vi "Engine Config Cluster to DSF Config File.vi"(8 "error in (no error)":errorcluster, 10 "dsf configuration file path":path, 11 "input cluster":T1) -> (0 "error out":errorcluster)   [LabVIEW 2017, in "Data Sharing Framework Core.lvlib" / "Data Sharing Framework Engine.lvlib"]
uses:
  Data Sharing Framework Engine.lvlib
  Configuration/1.0.0/Public/Controls/DSF Engine Framework Configuration.ctl
  Configuration/1.0.0/Public/Controls/DSF Engine Plugin Configuration.ctl
  Configuration/1.0.0/Public/Controls/DSF Timing Info.ctl
  Configuration/1.0.0/Public/Controls/DSF Engine Transfer Group Configuration.ctl
  Configuration/1.0.0/Public/Controls/DSF Direction.ctl
  Configuration/1.0.0/Public/Controls/DSF Engine Transfer Configuration.ctl
  Configuration/1.0.0/Public/Controls/DSF Byte Order.ctl
  Configuration/1.0.0/Public/Controls/DSF Engine Channel Configuration.ctl
  Configuration/1.0.0/Public/Controls/DSF Data Type.ctl
  Configuration/1.0.0/Public/Controls/DSF Settings Info.ctl
  Configuration/1.0.0/Public/Controls/DSF Plugin Info.ctl
  Configuration/1.0.0/Public/Controls/DSF Group Info.ctl
  Configuration/1.0.0/Public/Controls/DSF Transfer Info.ctl
  Configuration/1.0.0/Public/Controls/DSF Channel Info.ctl
  Configuration/1.0.0/Public/Write Item/Write Channel.vi
  Configuration/1.0.0/Public/Write Item/Write Transfer.vi
  Configuration/1.0.0/Public/Write Item/Write Group.vi
  Configuration/1.0.0/Public/Write Item/Write Plugin.vi
  Configuration/1.0.0/Data Sharing Framework Configuration.lvlib
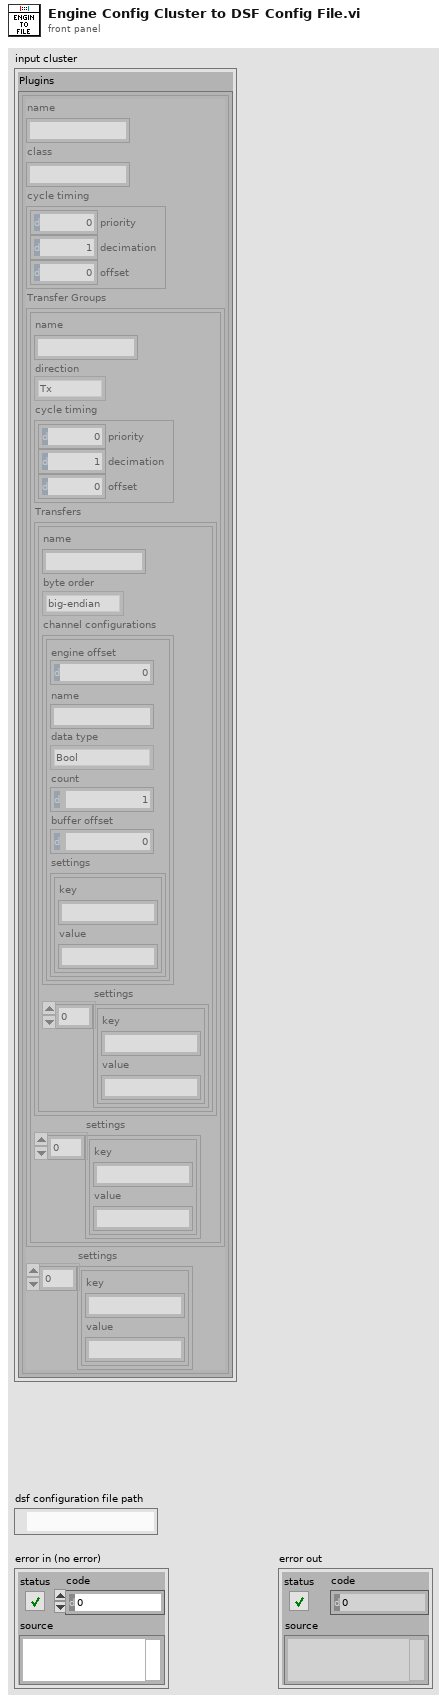
[diagram p1: front panel]
types:
  T1 = typedef "Data Sharing Framework Core.lvlib/Data Sharing Framework Configuration.lvlib/DSF Engine Framework Configuration.ctl" = cluster{"Plugins":T2[]}
  T2 = typedef "Data Sharing Framework Core.lvlib/Data Sharing Framework Configuration.lvlib/DSF Engine Plugin Configuration.ctl" = cluster{"name":string, "class":string, "cycle timing":T3, "Transfer Groups":T4[], "settings":T10}
  T3 = typedef "Data Sharing Framework Core.lvlib/Data Sharing Framework Configuration.lvlib/DSF Timing Info.ctl" = cluster{"priority":u64, "decimation":u64, "offset":u64}
  T4 = typedef "Data Sharing Framework Core.lvlib/Data Sharing Framework Configuration.lvlib/DSF Engine Transfer Group Configuration.ctl" = cluster{"name":string, "direction":T5, "cycle timing":T3, "Transfers":T6[], "settings":T10}
  T5 = typedef "Data Sharing Framework Core.lvlib/Data Sharing Framework Configuration.lvlib/DSF Direction.ctl" = enum8{"Tx", "Rx"}
  T6 = typedef "Data Sharing Framework Core.lvlib/Data Sharing Framework Configuration.lvlib/DSF Engine Transfer Configuration.ctl" = cluster{"name":string, "byte order":T7, "channel configurations":T8[], "settings":T10}
  T7 = typedef "Data Sharing Framework Core.lvlib/Data Sharing Framework Configuration.lvlib/DSF Byte Order.ctl" = enum8{"big-endian", "little-endian"}
  T8 = typedef "Data Sharing Framework Core.lvlib/Data Sharing Framework Configuration.lvlib/DSF Engine Channel Configuration.ctl" = cluster{"engine offset":u64, "name":string, "data type":T9, "count":u64, "buffer offset":u64, "settings":T10}
  T9 = typedef "Data Sharing Framework Core.lvlib/Data Sharing Framework Configuration.lvlib/DSF Data Type.ctl" = enum8{"Bool", "SGL", "DBL", "I8", "I16", "I32", "I64", "U8", "U16", "U32", "U64"}
  T10 = typedef "Data Sharing Framework Core.lvlib/Data Sharing Framework Configuration.lvlib/DSF Settings Info.ctl" = cluster{"key":string, "value":string}[]
  T11 = typedef "Data Sharing Framework Core.lvlib/Data Sharing Framework Configuration.lvlib/DSF Config Data RefNum.ctl" = refnum<k1>
  T12 = typedef "Data Sharing Framework Core.lvlib/Data Sharing Framework Configuration.lvlib/DSF Plugin Info.ctl" = cluster{"type":string, "timing":T3, "group ids":string[], "settings id":string}
  T13 = typedef "Data Sharing Framework Core.lvlib/Data Sharing Framework Configuration.lvlib/DSF Group Info.ctl" = cluster{"direction":T5, "timing":T3, "transfer ids":string[], "settings id":string}
  T14 = typedef "Data Sharing Framework Core.lvlib/Data Sharing Framework Configuration.lvlib/DSF Transfer Info.ctl" = cluster{"byte order":T7, "channel ids":string[], "settings id":string}
  T15 = typedef "Data Sharing Framework Core.lvlib/Data Sharing Framework Configuration.lvlib/DSF Channel Info.ctl" = cluster{"count":u64, "buffer offset":u64, "data type":T9, "settings id":string}
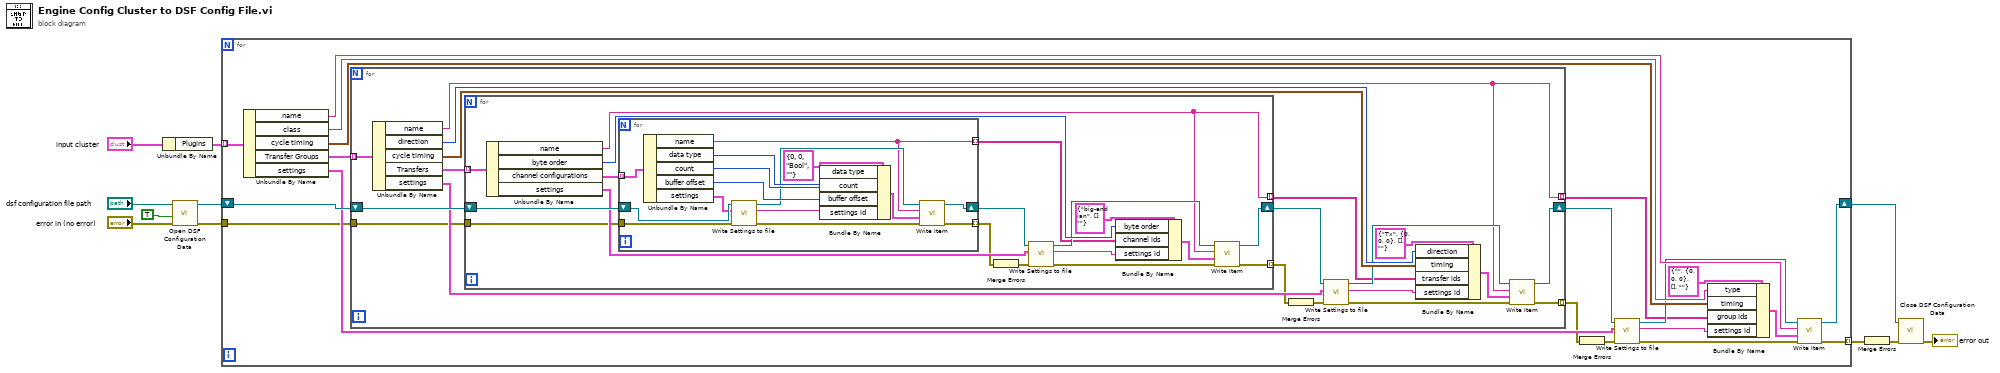
[diagram p0: block diagram]
diagram:
  n1 = Unbundle By Name("input cluster") -> ("Plugins"=w7:T2[])
  n2 = call "Open DSF Configuration Data.vi"("error in (no error)"="error in (no error)", "replace if found? (F)"=TRUE, "dsf configuration file path"="dsf configuration file path") -> ("error out"=w4:errorcluster, "dsf refnum"=w6:T11)  [unwired: 4 in, 3 out]
  n3 = for {
    tunnel: w7 -> [w30] mode=indexing
    shift-right: [w22] -> w5
    shift-left: w6 -> [w23]
    tunnel: w4 -> [w16]
    tunnel: [w13] -> w3 mode=indexing
    n4 = Unbundle By Name(w30) -> ("name"=w29:string, "class"=w26:string, "cycle timing"=w25:T3, "Transfer Groups"=w24:T4[], "settings"=w20:T10)
    n5 = for {
      tunnel: w24 -> [w49] mode=indexing
      shift-right: [w41] -> w18
      shift-left: w23 -> [w43]
      tunnel: [w36] -> w17 mode=indexing
      tunnel: w16 -> [w35]
      tunnel: [w34] -> w15 mode=indexing
      n6 = Unbundle By Name(w49) -> ("name"=w36:string, "direction"=w46:T5, "cycle timing"=w45:T3, "Transfers"=w44:T6[], "settings"=w39:T10)
      n7 = for {
        tunnel: w44 -> [w67] mode=indexing
        shift-right: [w60] -> w42
        shift-left: w43 -> [w62]
        tunnel: [w55] -> w37 mode=indexing
        tunnel: w35 -> [w54]
        tunnel: [w51] -> w33 mode=indexing
        n8 = Unbundle By Name(w67) -> ("name"=w55:string, "byte order"=w65:T7, "channel configurations"=w63:T8[], "settings"=w58:T10)
        n9 = for {
          tunnel: w63 -> [w82] mode=indexing
          shift-right: [w75] -> w61
          shift-left: w62 -> [w76]
          tunnel: [w71] -> w56 mode=indexing
          tunnel: w54 -> [w70]
          tunnel: [w68] -> w53 mode=indexing
          n10 = Unbundle By Name(w82) -> ("name"=w71:string, "data type"=w80:T9, "count"=w79:u64, "buffer offset"=w78:u64, "settings"=w73:T10)
          n11 = call "Write Settings to file.vi"("error in (no error)"=w70, "settings"=w73, "Refnum in"=w76) -> ("error out"=w69:errorcluster, "settings id"=w72:string, "Refnum out"=w74:T11)  [unwired: 6 in]
          n12 = Bundle By Name(cluster=T15 {"count"=0, "buffer offset"=0, "data type"=enum."Bool", "settings id"=""} ("values"), "data type"=w80, "count"=w79, "buffer offset"=w78, "settings id"=w72) -> (w77:T15)
          n13 = call-poly "Write Item.vi"("error in (no error)"=w69, "channel values"=w77, "id"=w71, "dsf refnum"=w74) -> ("error out"=w68:errorcluster, "dsf refnum out"=w75:T11)  [unwired: 5 in, 1 out]
        }
        n14 = Merge Errors(w53) -> (w50:errorcluster)
        n15 = call "Write Settings to file.vi"("error in (no error)"=w50, "settings"=w58, "Refnum in"=w61) -> ("error out"=w52:errorcluster, "settings id"=w57:string, "Refnum out"=w59:T11)  [unwired: 6 in]
        n16 = Bundle By Name(cluster=T14 {"byte order"=enum."big-endian", "channel ids"=[], "settings id"=""} ("values"), "byte order"=w65, "channel ids"=w56, "settings id"=w57) -> (w64:T14)
        n17 = call-poly "Write Item.vi"("error in (no error)"=w52, "transfer values"=w64, "id"=w55, "dsf refnum"=w59) -> ("error out"=w51:errorcluster, "dsf refnum out"=w60:T11)  [unwired: 5 in, 1 out]
      }
      n18 = Merge Errors(w33) -> (w31:errorcluster)
      n19 = call "Write Settings to file.vi"("error in (no error)"=w31, "settings"=w39, "Refnum in"=w42) -> ("error out"=w32:errorcluster, "settings id"=w38:string, "Refnum out"=w40:T11)  [unwired: 6 in]
      n20 = Bundle By Name(cluster=T13 {"direction"=enum."Tx", "timing"={"priority"=0, "decimation"=0, "offset"=0}, "transfer ids"=[], "settings id"=""} ("group values"), "direction"=w46, "timing"=w45, "transfer ids"=w37, "settings id"=w38) -> (w47:T13)
      n21 = call-poly "Write Item.vi"("error in (no error)"=w32, "group values"=w47, "id"=w36, "dsf refnum"=w40) -> ("error out"=w34:errorcluster, "dsf refnum out"=w41:T11)  [unwired: 5 in, 1 out]
    }
    n22 = Merge Errors(w15) -> (w12:errorcluster)
    n23 = call "Write Settings to file.vi"("error in (no error)"=w12, "settings"=w20, "Refnum in"=w18) -> ("error out"=w14:errorcluster, "settings id"=w21:string, "Refnum out"=w19:T11)  [unwired: 6 in]
    n24 = Bundle By Name(cluster=T12 {"type"="", "timing"={"priority"=0, "decimation"=0, "offset"=0}, "group ids"=[], "settings id"=""} ("plugin values"), "type"=w26, "timing"=w25, "group ids"=w17, "settings id"=w21) -> (w27:T12)
    n25 = call-poly "Write Item.vi"("error in (no error)"=w14, "plugin values"=w27, "id"=w29, "dsf refnum"=w19) -> ("error out"=w13:errorcluster, "dsf refnum out"=w22:T11)  [unwired: 5 in, 1 out]
  }
  n26 = Merge Errors(w3) -> (w1:errorcluster)
  n27 = call "Close DSF Configuration Data.vi"("error in (no error)"=w1, "dsf refnum"=w5) -> ("error out"=→"error out":errorcluster)  [unwired: 8 in, 1 out]
